vi "Speed Detector (FPGA).vi"(0 "Current In":fxp<+,14,6> format="%#_10g", 2 "CommSegs":i32, 11 "index In":i32) -> (4 "Speed Out":i32, 15 "index Out":i32)   [LabVIEW 2013]
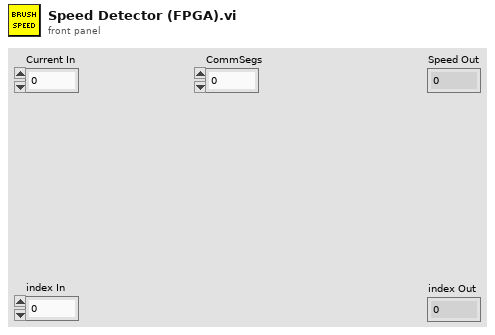
[diagram p1: front panel]
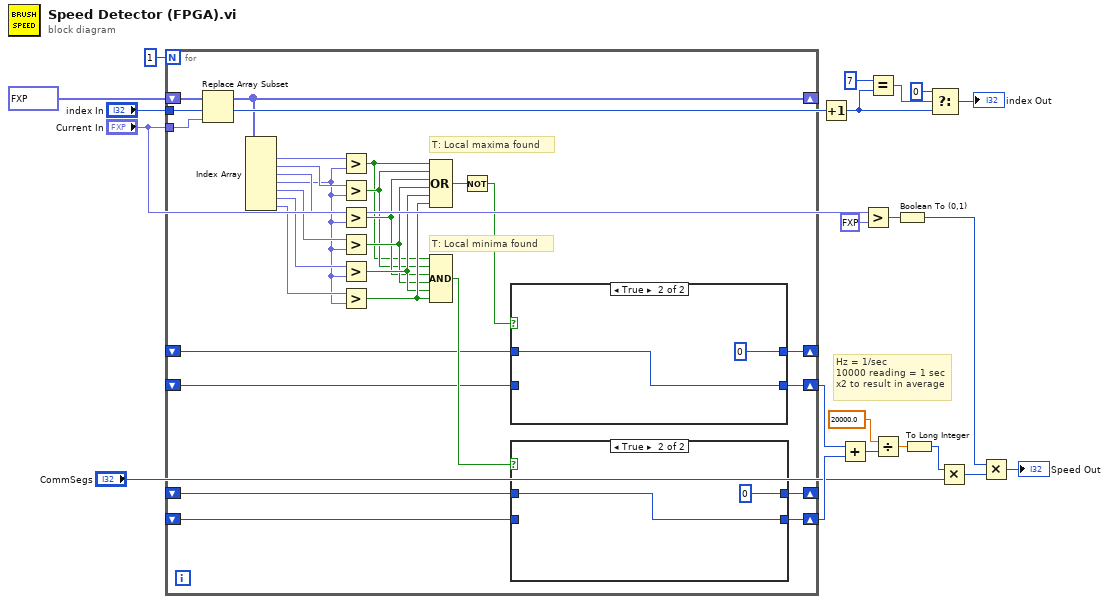
[diagram p0: block diagram]
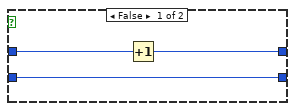
[diagram p2: hidden frame]
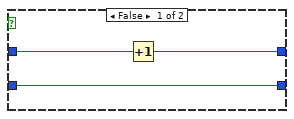
[diagram p3: hidden frame]
diagram:
  # "Hz = 1/sec\n10000 reading = 1 sec\nx2 to result in average"
  n1 = for {
    N: 1 -> [_]
    tunnel: "Current In" -> [w47]
    shift-right: [w46] -> _
    shift-left: fxp<+/-,24,5>[] [0.0, 0.0, 0.0, 0.0, 0.0, 0.0, 0.0] -> [w49]
    tunnel: "index In" -> [w48]
    shift-right: [w27] -> _
    shift-left: _ -> [w28]
    shift-right: [w26] -> _
    shift-left: _ -> [w29]
    shift-right: [w23] -> w13
    shift-left: _ -> [w22]
    shift-right: [w25] -> w12
    shift-left: _ -> [w24]
    # "T: Local maxima found"
    # "T: Local minima found"
    n2 = Replace Array Subset(array=w49, new element=w47, index=w48) -> (w46:fxp<+/-,24,5>[])
    n3 = Index Array(array=w46) -> (element #1=w45:fxp<+/-,24,5>, element #2=w43:fxp<+/-,24,5>, element #3=w44:fxp<+/-,24,5>, element #4=w39:fxp<+/-,24,5>, element #5=w42:fxp<+/-,24,5>, element #6=w41:fxp<+/-,24,5>, element #7=w40:fxp<+/-,24,5>)  [unwired: 7 in]
    n4 = Greater?(x=w45, y=w39) -> (0:w33:bool)
    n5 = Greater?(x=w43, y=w39) -> (0:w34:bool)
    n6 = Greater?(x=w44, y=w39) -> (0:w35:bool)
    n7 = Greater?(x=w42, y=w39) -> (0:w36:bool)
    n8 = Greater?(x=w41, y=w39) -> (0:w37:bool)
    n9 = Greater?(x=w40, y=w39) -> (0:w38:bool)
    n10 = Compound Arithmetic op=OR(w33, w34, w35, w36, w37, w38) -> (w32:bool)
    n11 = Compound Arithmetic op=AND(w33, w34, w35, w36, w37, w38) -> (w31:bool)
    n12 = Not(x=w32) -> (.not. x?=w30:bool)
    n13 = case shown="True" w30 {
      tunnel: w28 -> [w57 w58]
      tunnel: [w56 0] -> w27
      tunnel: [w55 w58] -> w23
      tunnel: w22 -> [w55 _]
      frame False {
        n14 = Increment(x=w57) -> (x+1=w56:i32)
      }
      frame True {
      }
    }
    n15 = case shown="True" w31 {
      tunnel: w29 -> [w51 w54]
      tunnel: [w50 0] -> w26
      tunnel: [w52 w54] -> w25
      tunnel: w24 -> [w52 _]
      frame False {
        n16 = Increment(x=w51) -> (x+1=w50:i32)
      }
      frame True {
      }
    }
  }
  n17 = Increment(x="index In") -> (x+1=w16:i32)
  n18 = Add(x=w13, y=w12) -> (x+y=w10:i32)
  n19 = Greater?(x="Current In", y=fxp<+,14,6> 1.0) -> (0:w4:bool)
  n20 = Equal?(x=7, y=w16) -> (x = y?=w17:bool)
  n21 = Divide(x=sgl 20000.0, y=w10) -> (x/y=w8:sgl)
  n22 = Boolean To (0,1)(Boolean=w4) -> (0, 1=w3:i16)
  n23 = To Long Integer(number=w8) -> (32bit integer=w7:i32)
  n24 = Select(t=0, s=w17, f=w16) -> (s? t:f=→"index Out":i32)
  n25 = Multiply(x=w7, y="CommSegs") -> (x*y=w2:i32)
  n26 = Multiply(x=w3, y=w2) -> (x*y=→"Speed Out":i32)
